vi "2D Plot Triangle.vi"(11 "appended array":dbl[](array[numeric])) -> (1 "Y":dbl[](array[numeric]), 2 "X":dbl[](array[numeric]), 3 "output cluster":cluster{dbl[], dbl[]})   [LabVIEW 2017]
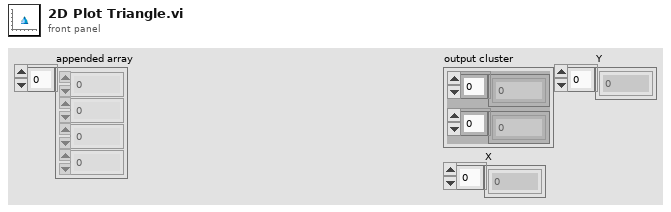
[diagram p1: front panel]
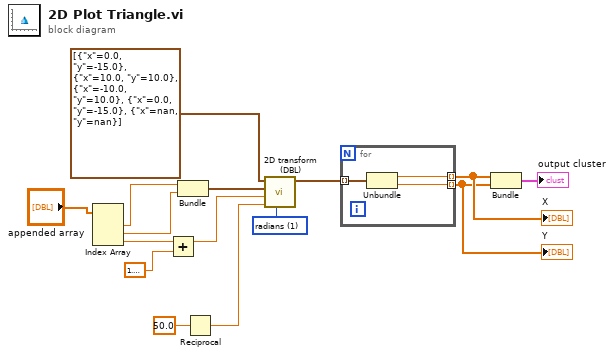
[diagram p0: block diagram]
diagram:
  w9 = u16 1 items=["degree", "radians"] ("angle unit")
  n1 = Index Array(array="appended array") -> (element #1=w13:dbl, element #2=w12:dbl, element #3=w10:dbl)  [unwired: 3 in]
  n2 = Add(x=w10, y=1.5707963267948966) -> (x+y=w2:dbl)
  n3 = Bundle(w13, w12) -> (w11:cluster{dbl, dbl})  [unwired: 1 in]
  n4 = Reciprocal(x=50.0 ("Scale")) -> (1/x=w7:dbl)
  n5 = call "2D transform (DBL).vi"("angle unit"=w9, "Scale"=w7, "Rotation Angle"=w2, "Translation"=w11, "line endpoints"=cluster{"x":dbl, "y":dbl}[] [{"x"=0.0, "y"=-15.0}, {"x"=10.0, "y"=10.0}, {"x"=-10.0, "y"=10.0}, {"x"=0.0, "y"=-15.0}, {"x"=nan, "y"=nan}]) -> ("tranformed line endpoint"=w6:cluster{"x":dbl, "y":dbl}[])  [unwired: 6 in]
  n6 = for {
    tunnel: w6 -> [w18] mode=indexing
    tunnel: [w17] -> w5 mode=indexing
    tunnel: [w16] -> w4 mode=indexing
    n7 = Unbundle(w18) -> ("x"=w17:dbl, "y"=w16:dbl)
  }
  "X" <- w5
  "Y" <- w4
  n8 = Bundle(w5, w4) -> (→"output cluster":cluster{dbl[], dbl[]})  [unwired: 1 in]
